vi "2004_FireEveryFiveMinutesInSpecificHour.vi"(8 "error in (no error)":errorcluster) -> (0 "error out":errorcluster)   [LabVIEW 2013]
uses:
  source/Cron.Jenkins/Cron.Jenkins.lvclass/Cron.Jenkins.ctl
  source/Cron.Jenkins/Write Job Name.vi
  <vilib>/addons/_JKI Toolkits/Caraya/classes/Assert/Assert True.vi
  source/Cron/Create Cron Expression.vi
  source/Cron/Compute Next Cron.vi
  source/Cron.Jenkins/Cron.Jenkins.lvclass
  <vilib>/addons/_JKI Toolkits/Caraya/classes/Test/Test.lvclass
  <vilib>/addons/_JKI Toolkits/Caraya/classes/Assert/Assert.lvclass
  source/openCron.lvlib
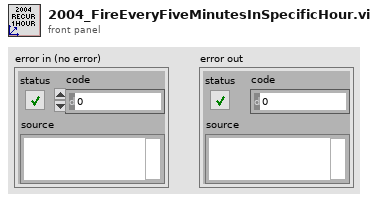
[diagram p1: front panel]
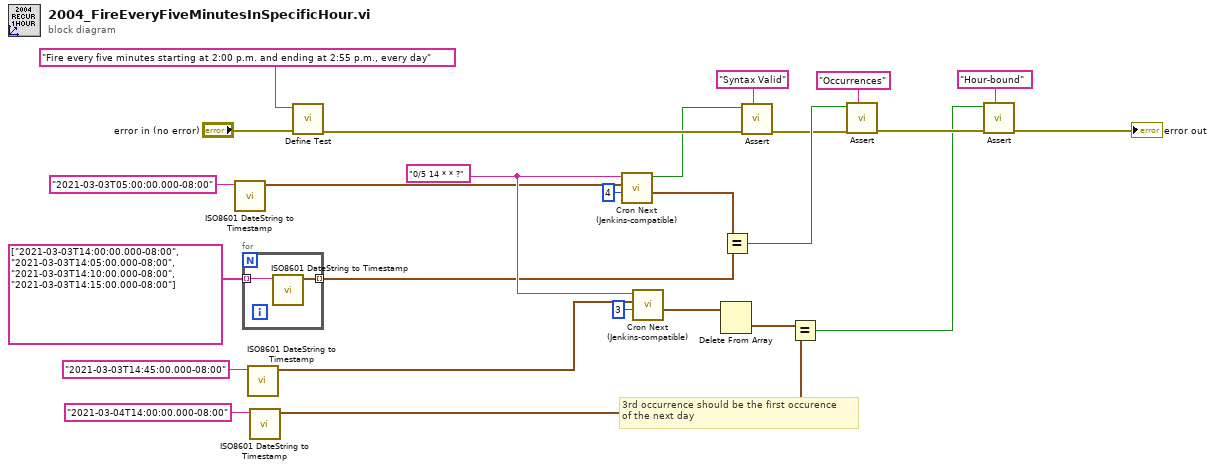
[diagram p0: block diagram]
diagram:
  w11 = "0/5 14 * * ?" ("Expression")
  # "3rd occurrence should be the first occurence\nof the next day"
  n1 = call <vilib>:"ISO8601 DateString to Timestamp.vi"("ISO8601 Date String"="2021-03-03T05:00:00.000-08:00" ("Expression")) -> ("Timestamp"=w4:timestamp)  [unwired: 8 in, 2 out]
  n2 = for {
    tunnel: string[] ["2021-03-03T14:00:00.000-08:00", "2021-03-03T14:05:00.000-08:00", "2021-03-03T14:10:00.000-08:00", "2021-03-03T14:15:00.000-08:00"] -> [w28] mode=indexing
    tunnel: [w27] -> w3 mode=indexing
    n3 = call <vilib>:"ISO8601 DateString to Timestamp.vi"("ISO8601 Date String"=w28) -> ("Timestamp"=w27:timestamp)  [unwired: 8 in, 2 out]
  }
  n4 = call <vilib>:"ISO8601 DateString to Timestamp.vi"("ISO8601 Date String"="2021-03-03T14:45:00.000-08:00" ("Expression")) -> ("Timestamp"=w5:timestamp)  [unwired: 8 in, 2 out]
  n5 = call <vilib>:"ISO8601 DateString to Timestamp.vi"("ISO8601 Date String"="2021-03-04T14:00:00.000-08:00" ("Expression")) -> ("Timestamp"=w1:timestamp)  [unwired: 8 in, 2 out]
  n6 = call <vilib>:"Define Test.vi"("error in (no error)"="error in (no error)", "Label (VI Title)"="Fire every five minutes starting at 2:00 p.m. and ending at 2:55 p.m., every day") -> ("error out"=w24:errorcluster)  [unwired: 8 in, 1 out]
  n7 = call "Cron Next (Jenkins-compatible).vi"("Nb Occurences (min: 1)"=u16 4, "Reference timestamp (Now)"=w4, "Cron Expression"=w11) -> ("Occurences"=w13:timestamp[], "syntax valid?"=w12:bool)  [unwired: 6 in, 1 out]
  n8 = call "Cron Next (Jenkins-compatible).vi"("Nb Occurences (min: 1)"=u16 3, "Reference timestamp (Now)"=w5, "Cron Expression"=w11) -> ("Occurences"=w9:timestamp[])  [unwired: 6 in, 2 out]
  n9 = Delete From Array(array=w9) -> (deleted portion=w15:timestamp)  [unwired: 2 in, 1 out]
  n10 = Equal?(x=w13, y=w3) -> (x = y?=w23:bool)
  n11 = call-poly <vilib>:"Assert.vi"("Label"="Syntax Valid" ("Label (VI Title)"), "error in (no error)"=w24, "True?"=w12) -> ("error out"=w22:errorcluster)  [unwired: 7 in, 1 out]
  n12 = Equal?(x=w15, y=w1) -> (x = y?=w16:bool)
  n13 = call-poly <vilib>:"Assert.vi"("Label"="Occurrences" ("Label (VI Title)"), "error in (no error)"=w22, "True?"=w23) -> ("error out"=w18:errorcluster)  [unwired: 7 in, 1 out]
  n14 = call-poly <vilib>:"Assert.vi"("Label"="Hour-bound" ("Label (VI Title)"), "error in (no error)"=w18, "True?"=w16) -> ("error out"=→"error out":errorcluster)  [unwired: 7 in, 1 out]
